vi "RigidField.vi"(10 "H":dbl[](array[numeric]), 11 "B":dbl[](array[numeric])) -> (1 "Br":dbl, 2 "Downward":dbl, 3 "Upward":dbl)   [LabVIEW 2019]
uses:
  <vilib>/gmath/NI_Gmath.lvlib
panel:
  out "error out":errorcluster
  out "Rigid Field":dbl
  out "array size":i32
  out "x 1":dbl[](array[numeric])
  out "y1":dbl[](array[numeric])
  out "x2":dbl[](array[numeric])
  out "y2":dbl[](array[numeric])
  out "XY Graph":cluster{"data":dbl[], "data":dbl[]}(graph)
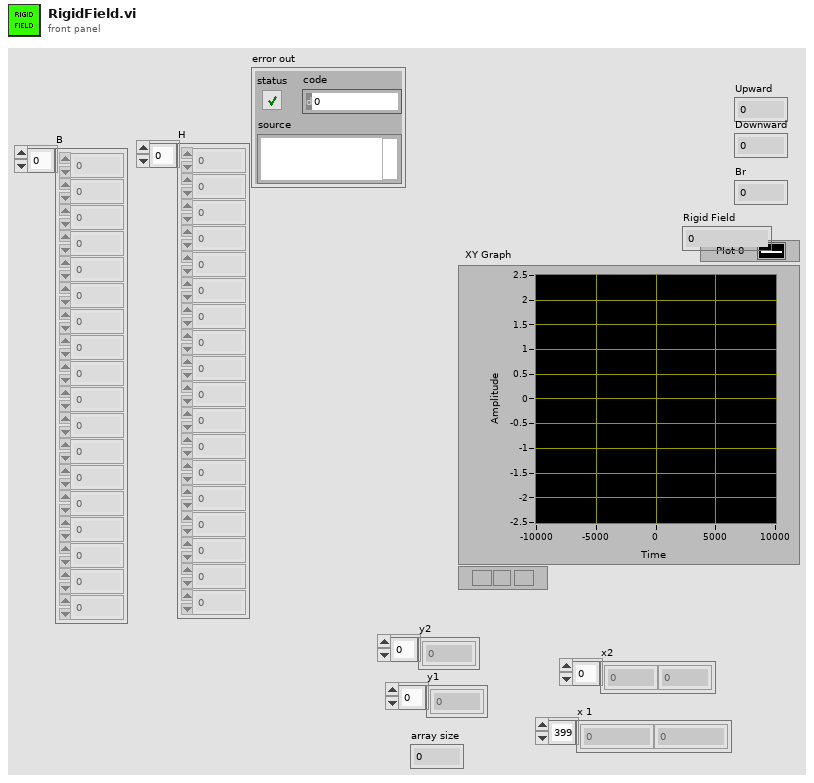
[diagram p1: front panel]
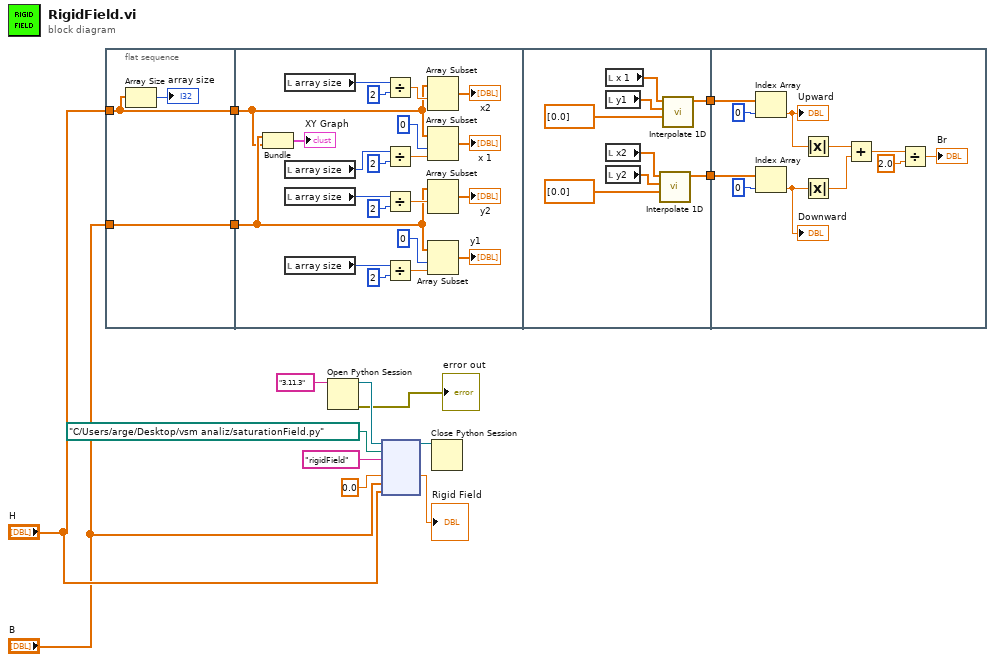
[diagram p0: block diagram]
diagram:
  n1 = flat-sequence {
    tunnel: "H" -> [w15]
    tunnel: "B" -> [w17]
    tunnel: [w17] -> w12
    tunnel: [w15] -> w11
    tunnel: w12 -> [w19]
    tunnel: w11 -> [w18]
    tunnel: [w40] -> w14
    tunnel: [w39] -> w13
    tunnel: w14 -> [w49]
    tunnel: w13 -> [w48]
    frame #0 {
      n2 = Array Size(array=w15) -> (size(s)=→"array size":i32)
    }
    frame #1 {
      n3 = Bundle("B"=w19, "H"=w18) -> (→"XY Graph":cluster{"B":dbl[], "H":dbl[]})  [unwired: 1 in]
      n4 = local read "array size"() -> (w30:i32)
      n5 = local read "array size"() -> (w22:i32)
      n6 = local read "array size"() -> (w35:i32)
      n7 = local read "array size"() -> (w27:i32)
      n8 = Divide(x=w30, y=2) -> (x/y=w32:dbl)
      n9 = Divide(x=w22, y=2) -> (x/y=w24:dbl)
      n10 = Divide(x=w35, y=2) -> (x/y=w33:dbl)
      n11 = Divide(x=w27, y=2) -> (x/y=w25:dbl)
      n12 = Array Subset(array=w18, index=w32) -> (→"x2":dbl[])  [unwired: 1 in]
      n13 = Array Subset(array=w18, index=0, length=w24) -> (→"x 1":dbl[])
      n14 = Array Subset(array=w19, index=w33) -> (→"y2":dbl[])  [unwired: 1 in]
      n15 = Array Subset(array=w19, index=0, length=w25) -> (→"y1":dbl[])
    }
    frame #2 {
      n16 = local read "x 1"() -> (w43:dbl[])
      n17 = local read "y1"() -> (w44:dbl[])
      n18 = local read "x2"() -> (w42:dbl[])
      n19 = local read "y2"() -> (w41:dbl[])
      n20 = call <vilib>:"Interpolate 1D.vi"("xi"=dbl[] [0.0], "X"=w41, "Y"=w42) -> ("yi"=w39:dbl[])  [unwired: 6 in, 2 out]
      n21 = call <vilib>:"Interpolate 1D.vi"("xi"=dbl[] [0.0], "X"=w44, "Y"=w43) -> ("yi"=w40:dbl[])  [unwired: 6 in, 2 out]
    }
    frame #3 {
      n22 = Index Array(array=w49, index=0) -> (element=w55:dbl)
      "Upward" <- w55
      n23 = Index Array(array=w48, index=0) -> (element=w47:dbl)
      "Downward" <- w47
      n24 = Absolute Value(x=w55) -> (abs(x)=w54:dbl)
      n25 = Absolute Value(x=w47) -> (abs(x)=w53:dbl)
      n26 = Add(x=w54, y=w53) -> (x+y=w52:dbl)
      n27 = Divide(x=w52, y=2.0) -> (x/y=→"Br":dbl)
    }
  }
  n28 = Open Python Session(python version="3.11.3" ("Python version")) -> (session out=w5:refnum<k35>, error out=→"error out":errorcluster)  [unwired: 2 in]
  n29 = node(w5, path "C:/Users/arge/Desktop/vsm analiz/saturationField.py" ("module path"), "rigidField" ("function name"), 0.0, "B", "H") -> (w10:refnum<k35>, →"Rigid Field":dbl)  [unwired: 3 in, 3 out]
  n30 = Close Python Session(session in=w10) -> ()  [unwired: 1 in, 1 out]
